vi "Two-Sided-Spectrum-To-One-Sided.vi"(10 "Block Size":i32=-1, 11 "waveform":waveform(dbl)) -> (2 "FFT- Phase":cluster{dbl, dbl, dbl[]}(graph), 3 "FFT- Mag":cluster{dbl, dbl, dbl[]}(graph))   [LabVIEW 2022 SP3]
uses:
  <vilib>/Analysis/2dsp.llb/Real FFT.vi
  <vilib>/Analysis/NI_AALPro.lvlib
panel:
  out "block size":dbl format="%0.2f"
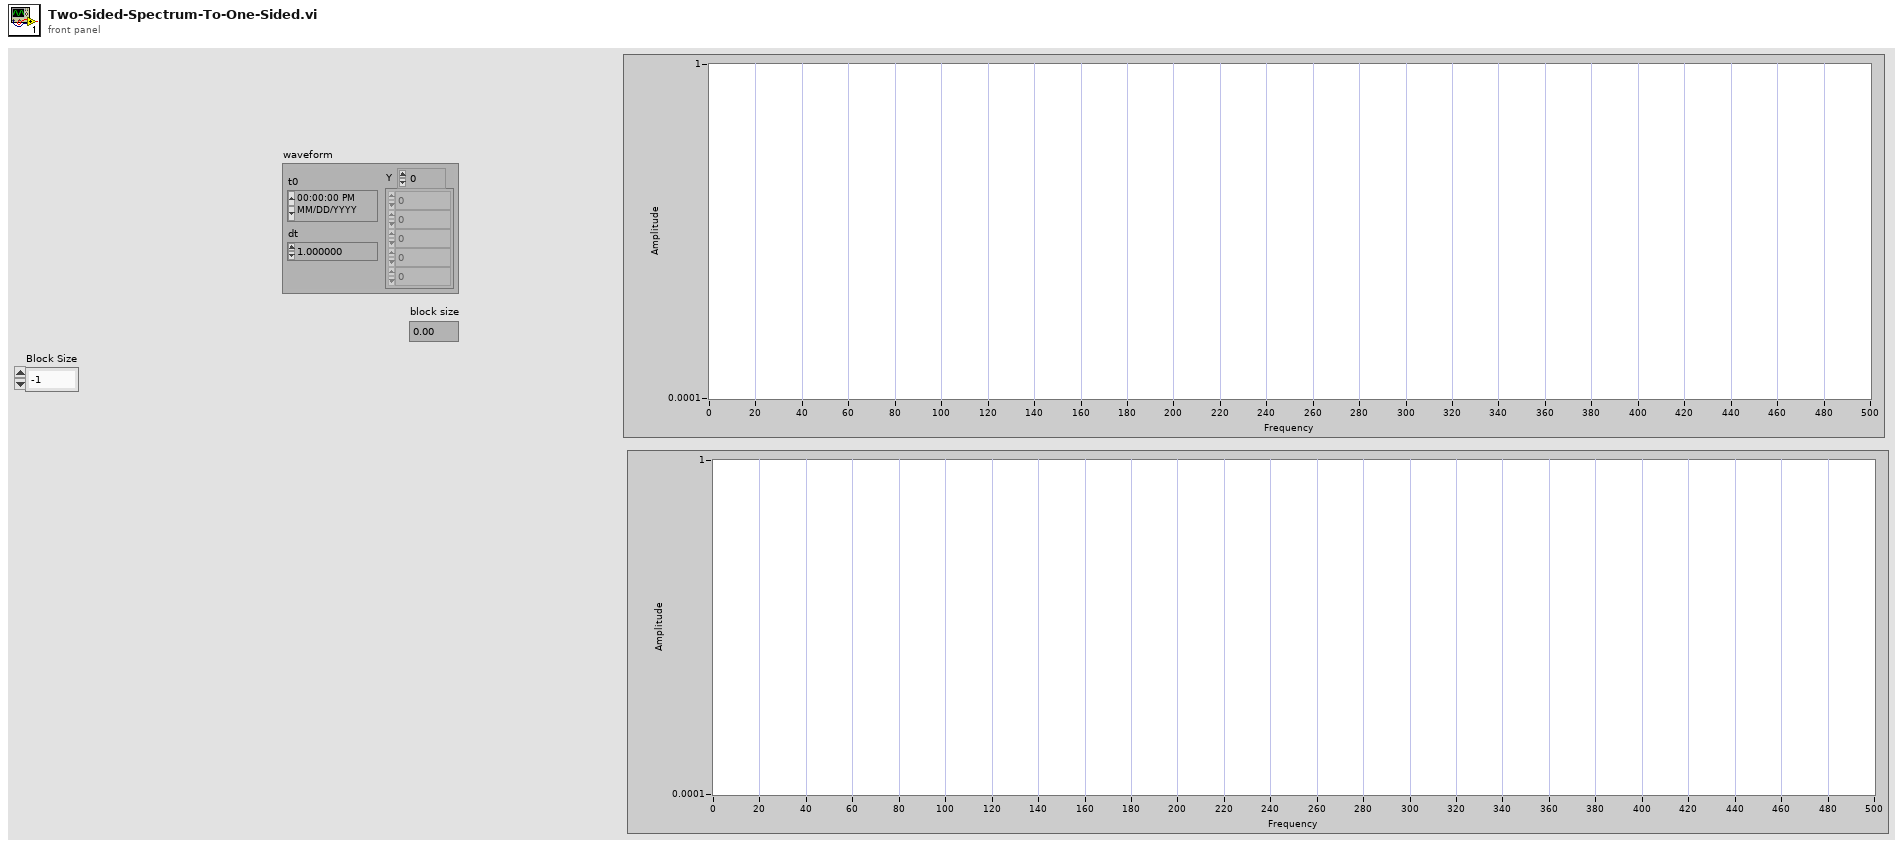
[diagram p1: front panel]
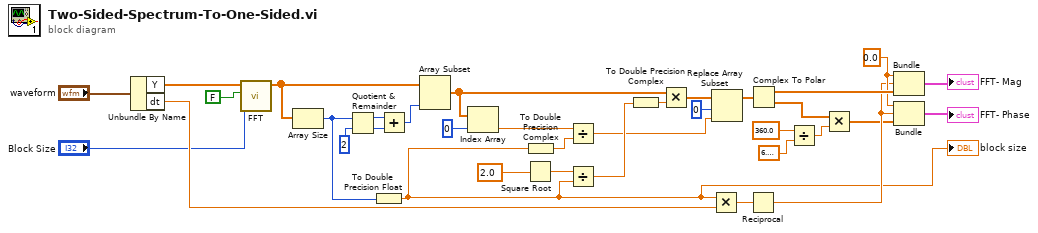
[diagram p0: block diagram]
diagram:
  w13 = 0.0
  n1 = Unbundle By Name("waveform") -> ("Y"=w18:dbl[], "dt"=w8:dbl)
  n2 = call-poly <vilib>:"FFT.vi"("FFT size"="Block Size", "shift?"=FALSE, "X"=w18) -> ("FFT {X}"=w20:cdb[])  [unwired: 7 in, 1 out]
  n3 = Array Size(array=w20) -> (size(s)=w26:i32)
  n4 = Quotient & Remainder(x=w26, y=2) -> (x-y*floor(x/y)=w32:i32, floor(x/y)=w31:i32)
  n5 = To Double Precision Float(number=w26) -> (double precision float=w7:dbl)
  "block size" <- w7
  n6 = Add(x=w32, y=w31) -> (x+y=w30:i32)
  n7 = Array Subset(array=w20, length=w30) -> (w25:cdb[])  [unwired: 1 in]
  n8 = Index Array(array=w25, index=0) -> (element=w22:cdb)
  n9 = Square Root(x=2.0) -> (sqrt(x)=w10:dbl)
  n10 = To Double Precision Complex(1:w7) -> (0:w9:cdb)
  n11 = Divide(x=w22, y=w9) -> (x/y=w21:cdb)
  n12 = Divide(x=w10, y=w7) -> (x/y=w27:dbl)
  n13 = To Double Precision Complex(1:w27) -> (0:w29:cdb)
  n14 = Multiply(x=w25, y=w29) -> (x*y=w28:cdb[])
  n15 = Multiply(x=w7, y=w8) -> (x*y=w17:dbl)
  n16 = Replace Array Subset(array=w28, new element=w21, index=0 ("Index")) -> (w19:cdb[])
  n17 = Reciprocal(x=w17) -> (1/x=w12:dbl)
  n18 = Complex To Polar(r * e^(i*theta)=w19) -> (r=w16:dbl[], theta=w2:dbl[])
  n19 = Divide(x=360.0, y=6.283185307179586) -> (x/y=w4:dbl)
  n20 = Multiply(x=w2, y=w4) -> (x*y=w1:dbl[])
  n21 = Bundle(w13, w12, w16) -> (→"FFT- Mag":cluster{dbl, dbl, dbl[]})  [unwired: 1 in]
  n22 = Bundle(w13, w12, w1) -> (→"FFT- Phase":cluster{dbl, dbl, dbl[]})  [unwired: 1 in]
